vi "Write observer.vi"(8 "error in (no error)":errorcluster, 10 "observer":string, 11 "Publisher in":refnum<class "Publisher.lvclass">) -> (0 "error out":errorcluster, 3 "Publisher out":refnum<class "Publisher.lvclass">)   [LabVIEW 2018, in "Publisher.lvclass"]
uses:
  Publisher.lvclass
  Publisher.lvclass/Publisher.ctl
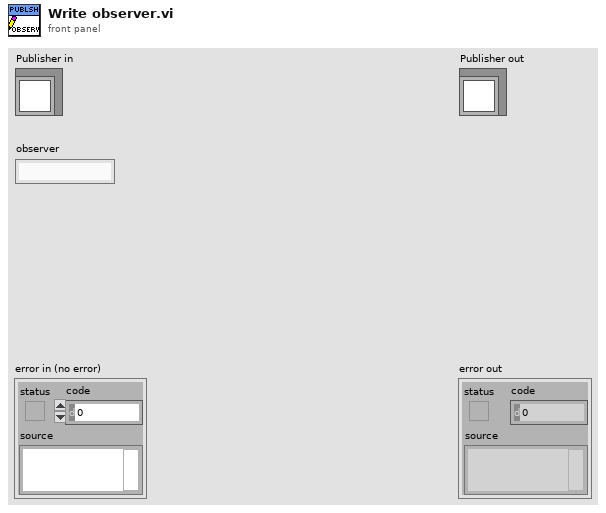
[diagram p1: front panel]
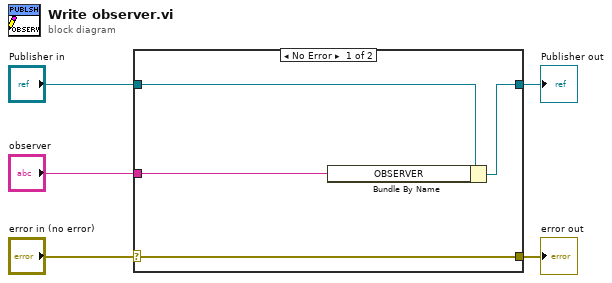
[diagram p0: block diagram]
diagram:
  n1 = case shown="No Error" "error in (no error)" {
    selector: "error in (no error)" -> [w9 w10]
    tunnel: [w9 w10] -> w4
    tunnel: [w7 w11] -> w2
    tunnel: "Publisher in" -> [w8 w11]
    tunnel: "observer" -> [w6 _]
    frame No Error {
      n2 = Bundle By Name(cluster=w8, "OBSERVER"=w6) -> (w7:refnum<class "Publisher.lvclass">)
    }
    frame Error {
    }
  }
  "error out" <- w4
  "Publisher out" <- w2
